vi "rate safety.vi"(2 "Max Rate":dbl=50.0, 3 "Desired Rate":dbl, 4 "Cutoff Rate":dbl=0.2, 5 "Encoder Rate":dbl) -> (0 "Output Rate":dbl, 1 "Encoder Rate Out":dbl)   [LabVIEW 2012]
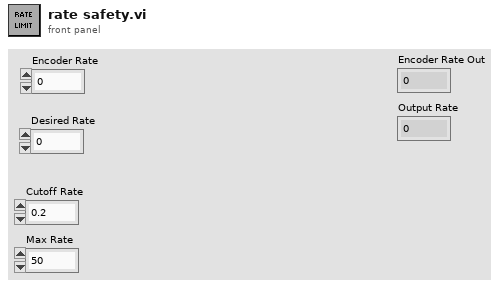
[diagram p1: front panel]
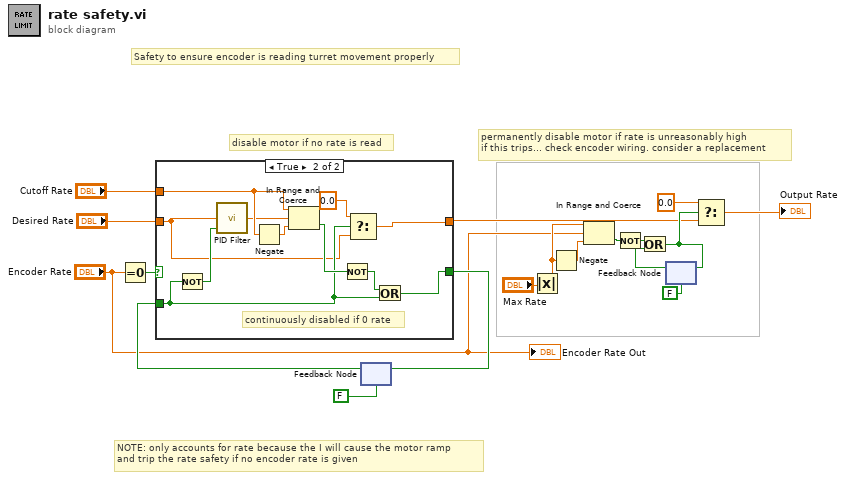
[diagram p0: block diagram]
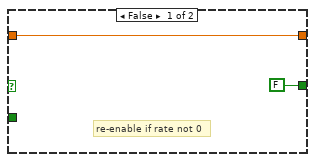
[diagram p2: hidden frame]
diagram:
  # "Safety to ensure encoder is reading turret movement properly"
  # "NOTE: only accounts for rate because the I will cause the motor ramp\nand trip the rate safety if no encoder rate is given"
  # "permanently disable motor if rate is unreasonably high\nif this trips... check encoder wiring. consider a replacement"
  # "disable motor if no rate is read"
  n1 = Equal To 0?(x="Encoder Rate") -> (x = 0?=w17:bool)
  n2 = feedback #1(FALSE ("x > y?")) -> (w10:bool)
  n3 = case shown="True" w17 {
    tunnel: "Desired Rate" -> [w20 w22]
    tunnel: [w20 w30] -> w7
    tunnel: [FALSE w27] -> w5
    tunnel: w10 -> [_ w26]
    tunnel: "Cutoff Rate" -> [_ w24]
    frame False {
      # "re-enable if rate not 0"
    }
    frame True {
      # "continuously disabled if 0 rate"
      n4 = Not(x=w26) -> (.not. x?=w23:bool)
      n5 = call "PID Filter.vi"("reinitialize? (F)"=w23, "input"=w22) -> ("output"=w21:dbl)  [unwired: 3 in]
      n6 = Negate(x=w24) -> (-x=w25:dbl)
      n7 = In Range and Coerce(upper limit=w24, x=w21, lower limit=w25) -> (In Range?=w29:bool)  [unwired: 1 out]
      n8 = Not(x=w29) -> (.not. x?=w28:bool)
      n9 = Select(t=0.0, s=w26, f=w22) -> (s? t:f=w30:dbl)
      n10 = Or(x=w28, y=w26) -> (x .or. y?=w27:bool)
    }
  }
  n11 = feedback-in #1(w5) -> ()
  n12 = Absolute Value(x="Max Rate") -> (abs(x)=w2:dbl)
  n13 = Negate(x=w2) -> (-x=w4:dbl)
  n14 = In Range and Coerce(upper limit=w2, x="Encoder Rate", lower limit=w4) -> (In Range?=w9:bool)  [unwired: 1 out]
  n15 = Not(x=w9) -> (.not. x?=w8:bool)
  n16 = feedback #2(FALSE ("x > y?")) -> (w14:bool)
  n17 = Or(x=w8, y=w14) -> (x .or. y?=w13:bool)
  n18 = feedback-in #2(w13) -> ()
  n19 = Select(t=0.0, s=w13, f=w7) -> (s? t:f=→"Output Rate":dbl)
  "Encoder Rate Out" <- "Encoder Rate"
